vi "Shared Variable Client - Variable API.vi"() -> ()   [LabVIEW 2014]
doc: "This client VI connects to Shared Variable Server.vi by using the Shared Variable API to read the server variable values."
panel:
  in  "Stop":bool
  in  "QN60KK30_BE01_Val":dbl
  # "Overview: Demonstrates the use of the Shared Variable API functions to read shared variable data from a server VI.\nRequirements: Windows\nInstructions:\n1. Make sure Shared Variable Server.vi is already running.\n2. Run this VI. It will read the values of the server shared variables through the Shared Variable API.\n3. Click Stop to stop the VI."
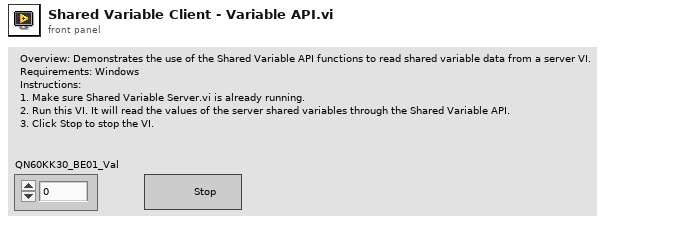
[diagram p1: front panel]
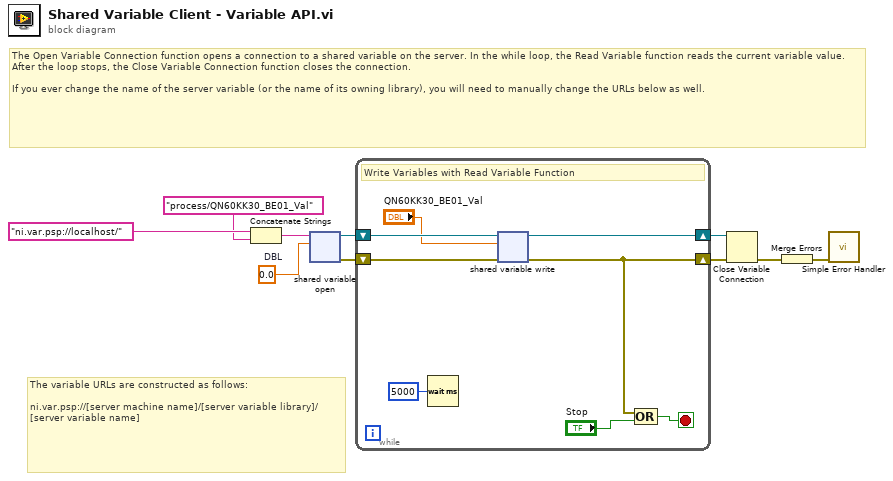
[diagram p0: block diagram]
diagram:
  w1 = 0.0  # DBL
  # "The Open Variable Connection function opens a connection to a shared variable on the server. In the while loop, the Read Variable function reads the current variable value. After the loop stops, the Close Variable Connection function closes the connection.\n\nIf you ever change the name of the server variable (or the name of its owning library), you will need to manually change the URLs below as well."
  # "The variable URLs are constructed as follows:\n\nni.var.psp://[server machine name]/[server variable library]/[server variable name]"
  n1 = Concatenate Strings("ni.var.psp://localhost/" ("string"), "process/QN60KK30_BE01_Val") -> (w2:string)
  n2 = shared-variable-open(w2, w1) -> (w7:refnum<k21>, w6:errorcluster)  [unwired: 2 in]
  n3 = while {
    shift-right: [w17] -> w5
    shift-left: w7 -> [w16]
    shift-right: [w12] -> w3
    shift-left: w6 -> [w15]
    stop <- w14 stop-if-true
    # "Write Variables with Read Variable Function"
    n4 = Wait (ms)(milliseconds to wait=u32 5000 ("millisecond multiple")) -> ()  [unwired: 1 out]
    n5 = shared-variable-write(w16, w15, "QN60KK30_BE01_Val") -> (w17:refnum<k21>, w12:errorcluster)
    n6 = Compound Arithmetic op=OR(w12, "Stop") -> (w14:bool)
  }
  n7 = Close Variable Connection(8:w3, 11:w5) -> (0:w4:errorcluster)
  n8 = Merge Errors(w4) -> (w8:errorcluster)
  n9 = call <vilib>:"Simple Error Handler.vi"("error in (no error)"=w8) -> ()  [unwired: 4 in, 5 out]
